vi "Open-Spec.vi"() -> (0 "error out":errorcluster, 2 "Number of Spectrometers":i32, 3 "Wrapper Out":u32)   [LabVIEW 2014]
doc: "Open Spectrometer\n\nAndré Romero - 2020\nandretec@ifsc.usp.br"
uses:
  Global variables.vi
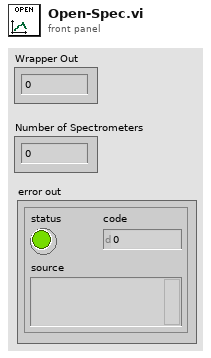
[diagram p1: front panel]
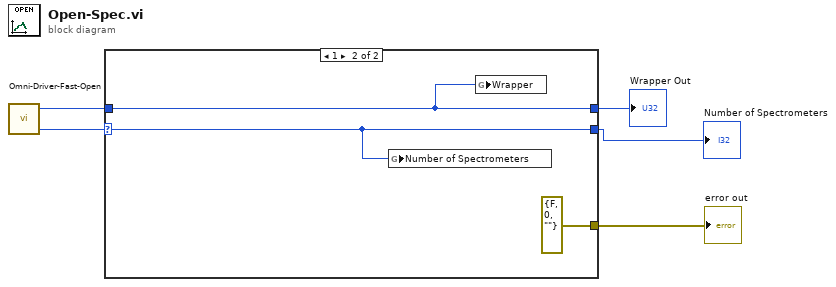
[diagram p0: block diagram]
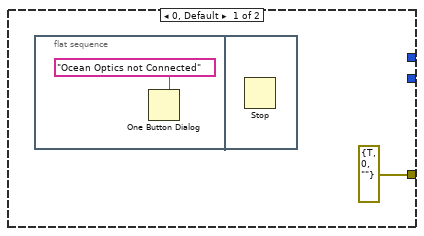
[diagram p2: hidden frame]
diagram:
  n1 = call "Omni-Driver-Fast-Open.vi"() -> ("Number of Spectrometers"=w2:i32, "Wrapper Out"=w3:u32)  [unwired: 4 in]
  n2 = case shown="1" w2 {
    selector: w2 -> [_ w9]
    tunnel: w3 -> [_ w10]
    tunnel: [_ w10] -> w4
    tunnel: [_ w9] -> w5
    tunnel: [errorcluster {"status"=TRUE, "code"=0, "source"=""} ("error constant") errorcluster {"status"=FALSE, "code"=0, "source"=""} ("error constant")] -> w1
    frame 0, Default {
      n3 = flat-sequence {
        frame #0 {
          n4 = One Button Dialog(message="Ocean Optics not Connected") -> ()  [unwired: 1 in, 1 out]
        }
        frame #1 {
          n5 = Stop() -> ()  [unwired: 1 in]
        }
      }
    }
    frame 1 {
      n6 = global write "Global variables.vi" "Number of Spectrometers"(w9) -> ()
      n7 = global write "Global variables.vi" "Wrapper"(w10) -> ()
    }
  }
  "Number of Spectrometers" <- w5
  "Wrapper Out" <- w4
  "error out" <- w1
